vi "BWC_CollectAnalogDataPtsAutomated.vi"() -> ()   [LabVIEW 2017]
uses:
  <vilib>/Utility/file.llb/Write Delimited Spreadsheet (DBL).vi
panel:
  out "XY Graph":cluster{"X":dbl, "Y":dbl}[](graph)=[{"X"=0.0, "Y"=0.6042307790041855}, {"X"=0.005, "Y"=0.6035980787723105}, {"X"=0.01, "Y"=0.6046155430476372}, {"X"=0.015, "Y"=0.6046361186649364}, {"X"=0.02, "Y"=0.604364520516617}, {"X"=0.025, "Y"=0.6062903982955967}, {"X"=0.030000000000000002, "Y"=0.6044962044673159}, {"X"=0.035, "Y"=0.6054807477549692}, {"X"=0.04, "Y"=0.6069498468299598}, {"X"=0.045, "Y"=0.6071123942066053}, {"X"=0.049999999999999996, "Y"=0.6049601846373598}, {"X"=0.05499999999999999, "Y"=0.6062410168140849}, {"X"=0.05999999999999999, "Y"=0.608494046908086}, {"X"=0.06499999999999999, "Y"=0.6094004028500115}, {"X"=0.06999999999999999, "Y"=0.6050311705170327}, {"X"=0.075, "Y"=0.6072564235276825}, {"X"=0.08, "Y"=0.6058830010731222}, {"X"=0.085, "Y"=0.6069652785429327}, {"X"=0.09000000000000001, "Y"=0.6077008568612928}, {"X"=0.09500000000000001, "Y"=0.6063922476012168}, {"X"=0.10000000000000002, "Y"=0.6082502258431176}, {"X"=0.10500000000000002, "Y"=0.6087615299329465}, {"X"=0.11000000000000003, "Y"=0.6087450694391063}, {"X"=0.11500000000000003, "Y"=0.6086936303958649}, {"X"=0.12000000000000004, "Y"=0.6072842006110344}, {"X"=0.12500000000000003, "Y"=0.6104528456747436}, {"X"=0.13000000000000003, "Y"=0.6093520501493626}, {"X"=0.13500000000000004, "Y"=0.6090310705195342}, {"X"=0.14000000000000004, "Y"=0.6108839048571113}, {"X"=0.14500000000000005, "Y"=0.6091555530041793}]
  out "error out":errorcluster={"status"=TRUE, "code"=43, "source"="Open/Create/Replace File in Write Spreadsheet String.vi->Write Delimited Spreadsheet (DBL).vi->BWC_CollectAnalogDataPtsAutomated.vi"}
  out "Error Out":errorcluster
  in  "NextAngle":dbl
  in  "angle/mean/std/num":dbl[][](array[numeric])=[[0.0, 0.6042307790041855, 0.19994807313898835, 40001.0], [0.005, 0.6035980787723105, 0.19970499180431311, 40001.0], [0.01, 0.6046155430476372, 0.199713086326253, 40001.0], [0.015, 0.6046361186649364, 0.19940124576393548, 40001.0], [0.02, 0.604364520516617, 0.19927380846502085, 40001.0], [0.025, 0.6062903982955967, 0.1987938986580054, 40001.0], [0.030000000000000002, 0.6044962044673159, 0.19886077875522098, 40001.0], [0.035, 0.6054807477549692, 0.19973524990707656, 40001.0], [0.04, 0.6069498468299598, 0.1994013496834136, 40001.0], [0.045, 0.6071123942066053, 0.199313293161399, 40001.0], [0.049999999999999996, 0.6049601846373598, 0.1994857483130004, 40001.0], [0.05499999999999999, 0.6062410168140849, 0.19966923858279817, 40001.0], [0.05999999999999999, 0.608494046908086, 0.20043486981994663, 40001.0], [0.06499999999999999, 0.6094004028500115, 0.2007617921532046, 40001.0], [0.06999999999999999, 0.6050311705170327, 0.19962346286144142, 40001.0], [0.075, 0.6072564235276825, 0.20046115684365937, 40001.0], [0.08, 0.6058830010731222, 0.20008527207371796, 40001.0], [0.085, 0.6069652785429327, 0.19993214656760383, 40001.0], [0.09000000000000001, 0.6077008568612928, 0.20038234883741932, 40001.0], [0.09500000000000001, 0.6063922476012168, 0.1993924789434216, 40001.0], [0.10000000000000002, 0.6082502258431176, 0.20012860172637706, 40001.0], [0.10500000000000002, 0.6087615299329465, 0.20159195822590326, 40001.0], [0.11000000000000003, 0.6087450694391063, 0.1993806767993975, 40001.0], [0.11500000000000003, 0.6086936303958649, 0.20126433387910456, 40001.0], [0.12000000000000004, 0.6072842006110344, 0.20035512036281494, 40001.0], [0.12500000000000003, 0.6104528456747436, 0.20050443038279972, 40001.0], [0.13000000000000003, 0.6093520501493626, 0.20183789637385943, 40001.0], [0.13500000000000004, 0.6090310705195342, 0.20100460954737798, 40001.0], [0.14000000000000004, 0.6108839048571113, 0.20092057934371635, 40001.0], [0.14500000000000005, 0.6091555530041793, 0.2012493360977225, 40001.0]]
  in  "Acquisition Time (s)":dbl=2.0 caption="Acquisition Time (s) (no change)"
  in  "stepSize":dbl=0.005
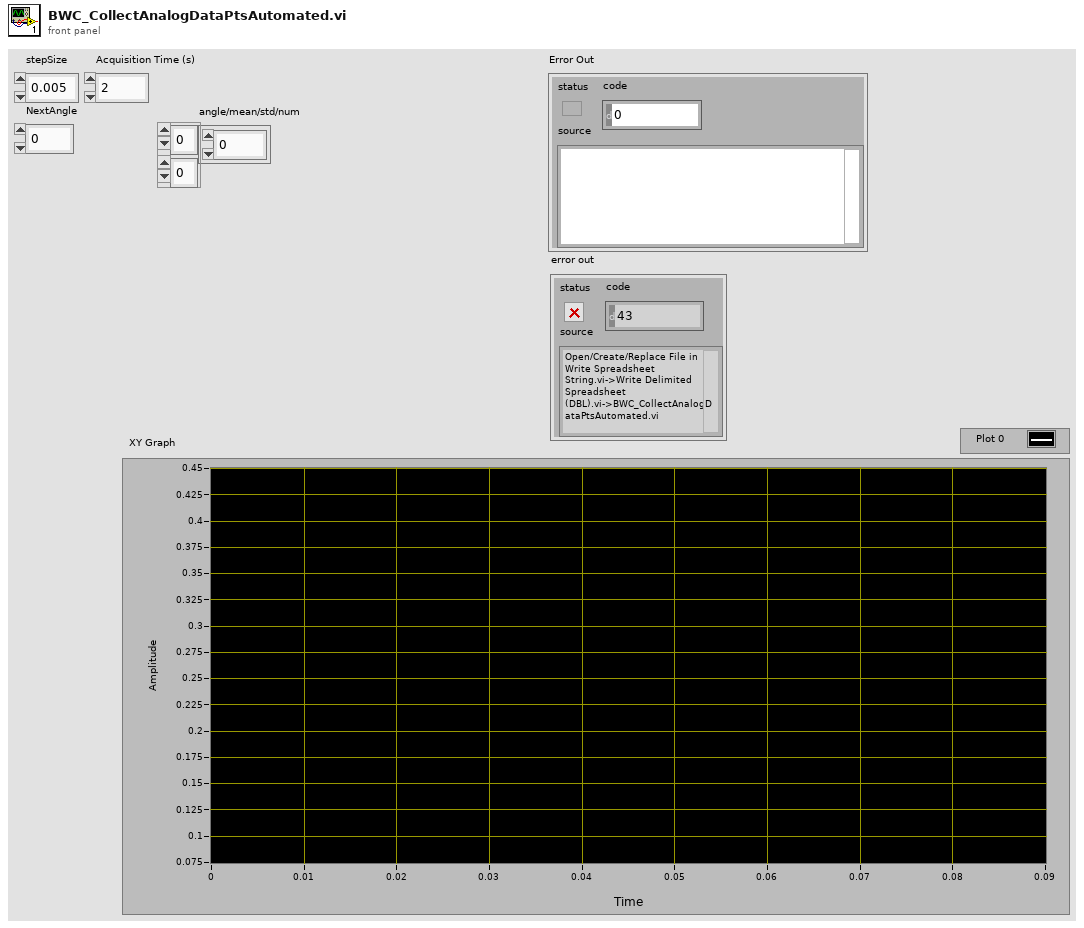
[diagram p1: front panel]
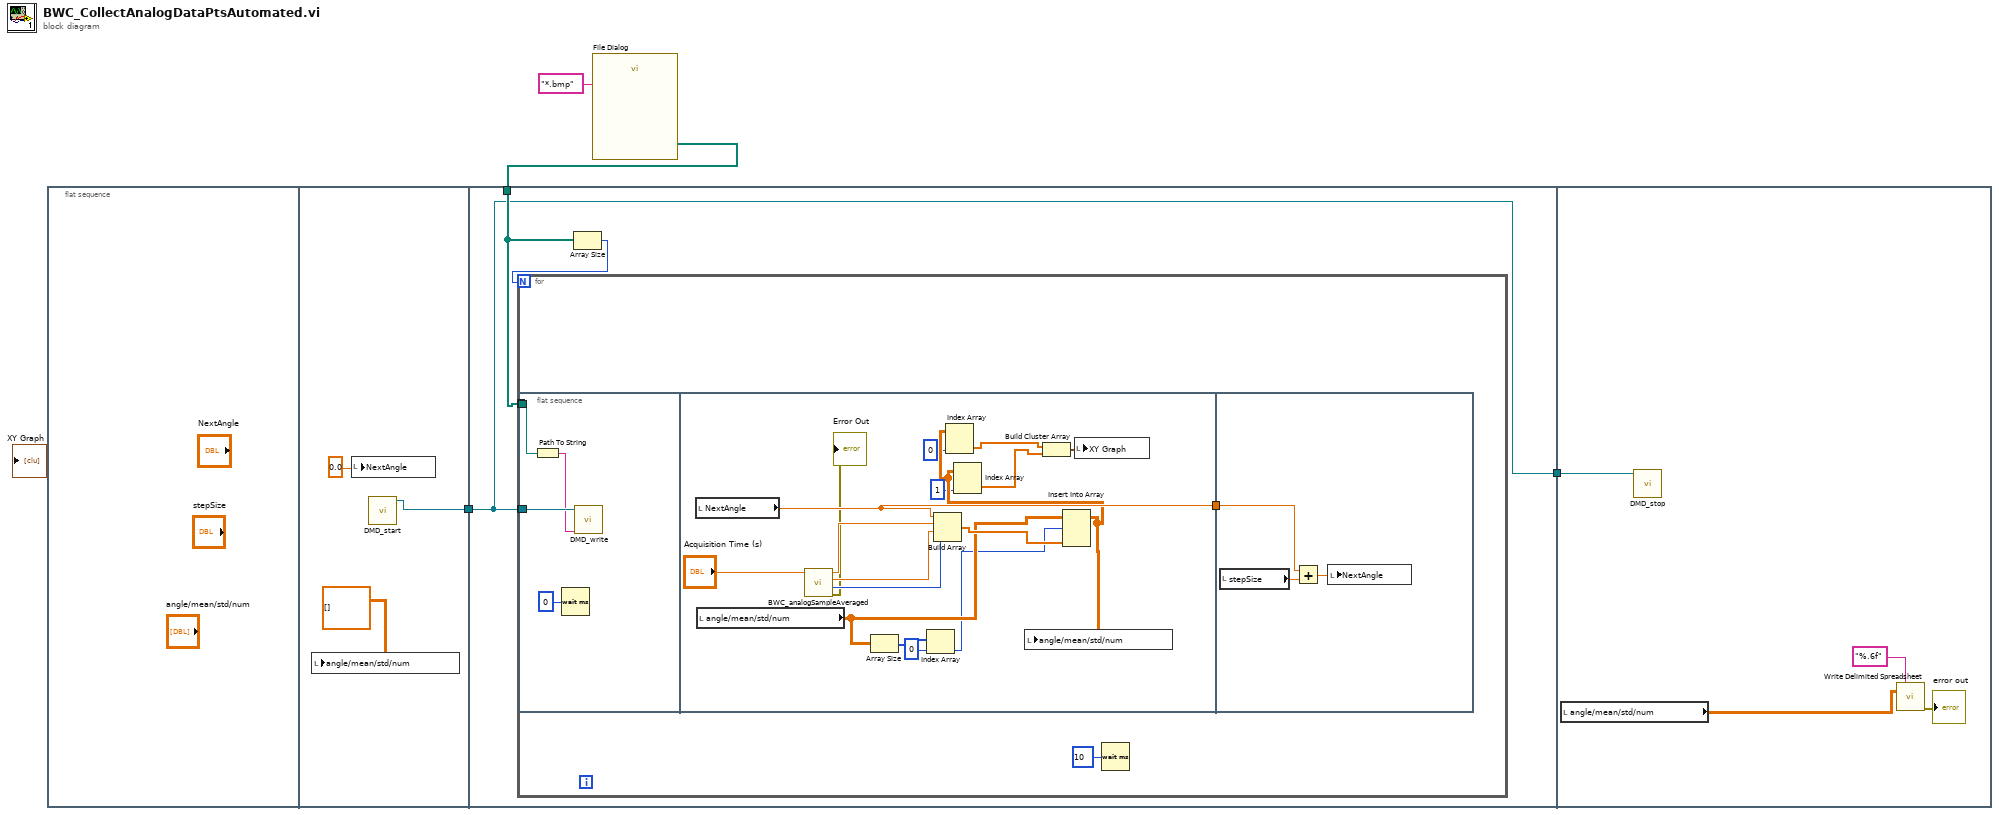
[diagram p0: block diagram]
diagram:
  n1 = flat-sequence {
    tunnel: [w5] -> w2
    tunnel: w3 -> [w10]
    tunnel: w2 -> [w8]
    tunnel: [w8] -> w1
    tunnel: w1 -> [w39]
    frame #0 {
    }
    frame #1 {
      n2 = local write "angle/mean/std/num"(dbl[][] []) -> ()
      n3 = local write "NextAngle"(0.0 ("NextAngle")) -> ()
      n4 = call "DMD_start.vi"() -> ("reference out"=w5:refnum<k24>)  [unwired: 10 in, 1 out]
    }
    frame #2 {
      n5 = Array Size(array=w10) -> (size(s)=w9:i32)
      n6 = for {
        N: w9 -> [_]
        tunnel: w10 -> [w11] mode=indexing
        tunnel: w8 -> [w12]
        n7 = flat-sequence {
          tunnel: w12 -> [w18]
          tunnel: w11 -> [w17]
          tunnel: [w26] -> w13
          tunnel: w13 -> [w37]
          frame #0 {
            n8 = Path To String(path=w17) -> (string=w16:string)
            n9 = Wait (ms)(milliseconds to wait=u32 0) -> ()  [unwired: 1 out]
            n10 = call "DMD_write.vi"("String"=w16, "reference out"=w18) -> ()  [unwired: 9 in, 1 out]
          }
          frame #1 {
            n11 = local read "NextAngle"() -> (w26:dbl)
            n12 = local read "angle/mean/std/num"() -> (w30:dbl[][])
            n13 = call "BWC_analogSampleAveraged.vi"("Acquisition Time (s)"="Acquisition Time (s)") -> ("Error Out"=→"Error Out":errorcluster, "size(s)"=w32:i32, "standard deviation"=w33:dbl, "mean"=w34:dbl)  [unwired: 7 in]
            n14 = Array Size(array=w30) -> (size(s)=w29:i32[])
            n15 = Index Array(array=w29, index=0) -> (element=w27:i32)
            n16 = Build Array(w26, w34, w33, w32) -> (w31:dbl[])
            n17 = Insert Into Array(array=w30, index (row)=w27, new element=w31) -> (w24:dbl[][])  [unwired: 1 in]
            n18 = Index Array(array=w24, index (col)=0 ("disabled index (col)")) -> (element=w21:dbl[])  [unwired: 1 in]
            n19 = Index Array(array=w24, index (col)=1 ("disabled index (col)")) -> (element=w20:dbl[])  [unwired: 1 in]
            n20 = local write "angle/mean/std/num"(w24) -> ()
            n21 = Build Cluster Array(w21, w20) -> (w19:cluster{dbl, dbl}[])
            n22 = local write "XY Graph"(w19) -> ()
          }
          frame #2 {
            n23 = local read "stepSize"() -> (w38:dbl)
            n24 = Add(x=w37, y=w38) -> (x+y=w36:dbl)
            n25 = local write "NextAngle"(w36) -> ()
          }
        }
        n26 = Wait (ms)(milliseconds to wait=u32 10) -> ()  [unwired: 1 out]
      }
    }
    frame #3 {
      n27 = local read "angle/mean/std/num"() -> (w42:dbl[][])
      n28 = call "DMD_stop.vi"("reference out"=w39) -> ()  [unwired: 10 in, 1 out]
      n29 = call-poly <vilib>:"Write Delimited Spreadsheet.vi"("format (%.3f)"="%.6f", "2D data"=w42) -> ("error out"=→"error out":errorcluster)  [unwired: 12 in, 1 out]
    }
  }
  n30 = call "File Dialog"("pattern (all files)"="*.bmp") -> ("selected paths"=w3:path[])  [unwired: 11 in, 3 out]
